vi "Update VI List.vi"(8 "error in (no error)":errorcluster, 10 "VI Infomation":T1[](array[typedef]), 11 "Interface in":refnum<class "Interface.lvclass">) -> (0 "error out":errorcluster, 3 "Interface out":refnum<class "Interface.lvclass">)   [LabVIEW 2015, in "Interface.lvlib" / "Interface.lvclass"]
uses:
  Interface.lvclass
  Controls/VI Infomation.ctl
  Interface.lvlib
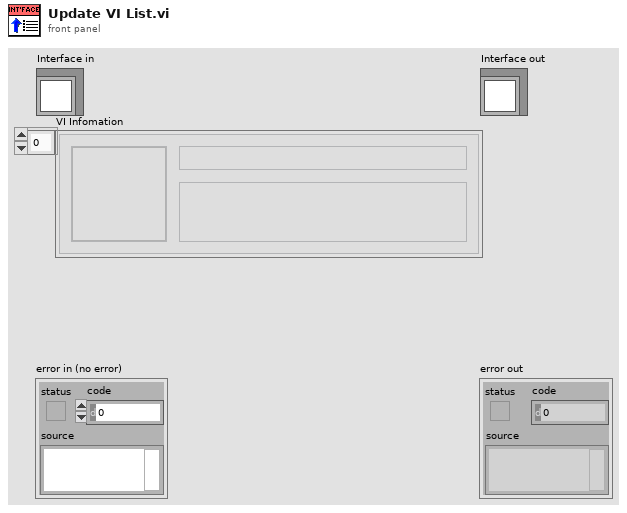
[diagram p1: front panel]
types:
  T1 = typedef "Interface.lvlib/VI Infomation.ctl" = cluster{"VI Name":string, "VI Description":string, "VI Icon":picture}
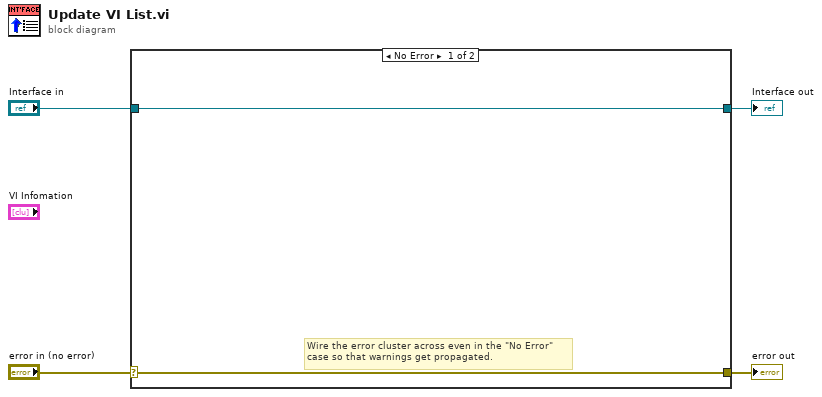
[diagram p0: block diagram]
diagram:
  n1 = case shown="No Error" "error in (no error)" {
    selector: "error in (no error)" -> [w5 w8]
    tunnel: [w5 w8] -> w3
    tunnel: [w6 w7] -> w1
    tunnel: "Interface in" -> [w6 w7]
    frame No Error {
      # "Wire the error cluster across even in the \"No Error\"\ncase so that warnings get propagated."
    }
    frame Error {
    }
  }
  "error out" <- w3
  "Interface out" <- w1
